vi "Variant to JSONRPC result .vi"(8 "error in (no error)":errorcluster, 11 "variant":variant) -> (0 "error out":errorcluster, 3 "<JSON>":string)   [LabVIEW 2019, in "JSON-RPC.lvlib"]
uses:
  JSON-RPC.lvlib
  <vilib>/Utility/Data Type/NI_Data Type.lvlib
  <vilib>/JDP Science/JSONtext/JSONtext.lvlib
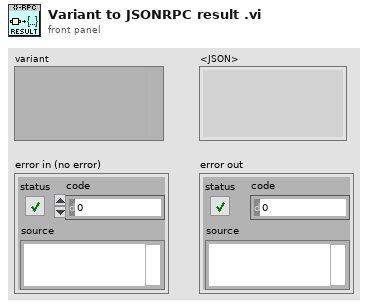
[diagram p1: front panel]
types:
  T1 = typedef "JSONtext.lvlib/JSON Value Type.ctl" = enum16{"Not a JSON Value", "JSON Object", "JSON Array", "String", "Number", "true", "false", "null"}
  T2 = typedef "NI_Data Type.lvlib/Data Type.ctl" = enum8{"Invalid Type", "Void", "I8", "I16", "I32", "I64", "U8", "U16", "U32", "U64", "Single Float", "Double Float", "Extended Float", "Single Complex", "Double Complex", "Extended Complex", "Enum U8", "Enum U16", "Enum U32", "Enum U64", "Single Float With Unit", "Double Float With Unit", "Extended Float With Unit", "Single Complex with Unit", "Double Complex with Unit", "Extended Complex with Unit", "Boolean", "String", "Path", "Picture", "Tag", "Array", "Cluster", "Variant", "LV Variant", "Waveform", "Timestamp", "Digital Waveform", "Digital Data", "ExpressData", "Refnum", "External Data", "VI", "Poly VI", "LabVIEW Class Instance", "Fixed Point", "Set Collection", "Map Collection"}
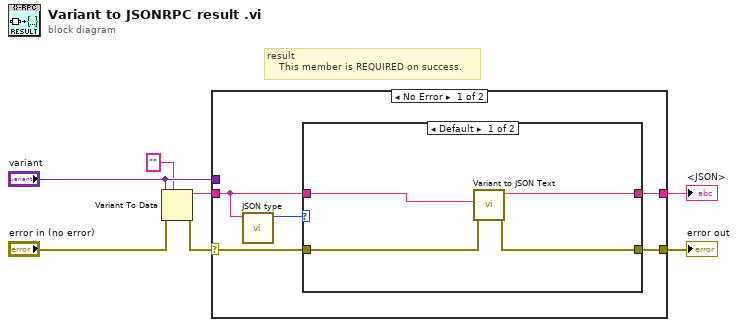
[diagram p0: block diagram]
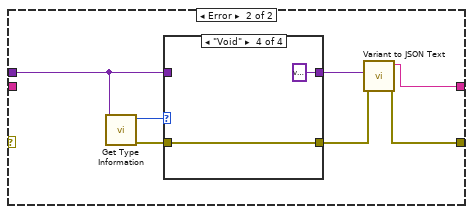
[diagram p3: hidden frame]
diagram:
  # "result\n    This member is REQUIRED on success."
  n1 = Variant To Data(error in="error in (no error)", type="", Variant="variant") -> (data=w3:string, error out=w1:errorcluster)
  n2 = case shown="No Error" w1 {
    selector: w1 -> [w9 _]
    tunnel: [w8 w25] -> w7
    tunnel: [w11 w24] -> w6
    tunnel: "variant" -> [_ w23]
    tunnel: w3 -> [w10 _]
    frame No Error {
      n3 = call <vilib>:"JSON type.vi"("JSON"=w10) -> ("JSON Value Type"=w12:T1)  [unwired: 9 in, 1 out]
      n4 = case shown="Default" w12 {
        tunnel: [w16 w18] -> w11
        tunnel: w10 -> [w13 w18]
        tunnel: w9 -> [w15 w17]
        tunnel: [w14 w17] -> w8
        frame Default {
          n5 = call <vilib>:"Variant to JSON Text.vi"("error in (no error)"=w15, "Variant"=w13) -> ("error out"=w14:errorcluster, "<JSON>"=w16:string)  [unwired: 7 in, 1 out]
        }
        frame "JSON Object", "JSON Array" {
        }
      }
    }
    frame Error {
      n6 = call <vilib>:"Get Type Information.vi"("variant"=w23) -> ("error out"=w20:errorcluster, "type"=w19:T2)  [unwired: 6 in, 3 out]
      n7 = case shown="\"Void\"" w19 {
        tunnel: w23 -> [w26 w28 w31 _]
        tunnel: [w26 w28 w31 variant ("params")] -> w21
        tunnel: w20 -> [w27 w29 w30 w32]
        tunnel: [w27 w29 w30 w32] -> w22
        frame Default {
        }
        frame "Cluster" {
        }
        frame "Array" {
        }
        frame "Void" {
        }
      }
      n8 = call <vilib>:"Variant to JSON Text.vi"("error in (no error)"=w22, "Variant"=w21) -> ("error out"=w25:errorcluster, "<JSON>"=w24:string)  [unwired: 7 in, 1 out]
    }
  }
  "error out" <- w7
  "<JSON>" <- w6
